vi "客户端侦听列表.vi"() -> ()   [LabVIEW 2016, in "wxpusher.lvlib"]
uses:
  wxpusher.lvlib
  <vilib>/Utility/miscctls.llb/LVPointTypeDef.ctl
  <vilib>/httpClient/LabVIEWHTTPClient.lvlib
panel:
  out "回调时间":timestamp
  out "有效主机列表":T1(array[cluster])
  out "长度":i32
  out "现场主机回调信息":string
  in  "开机启动":bool
  out "remote port":u16
  out "remote address":string
  out "服务器回调信息源码":string
  out "回调信息":T2
  out "新增主机列表":T1(array[cluster])
  in  "客户端列表":i32(listbox)
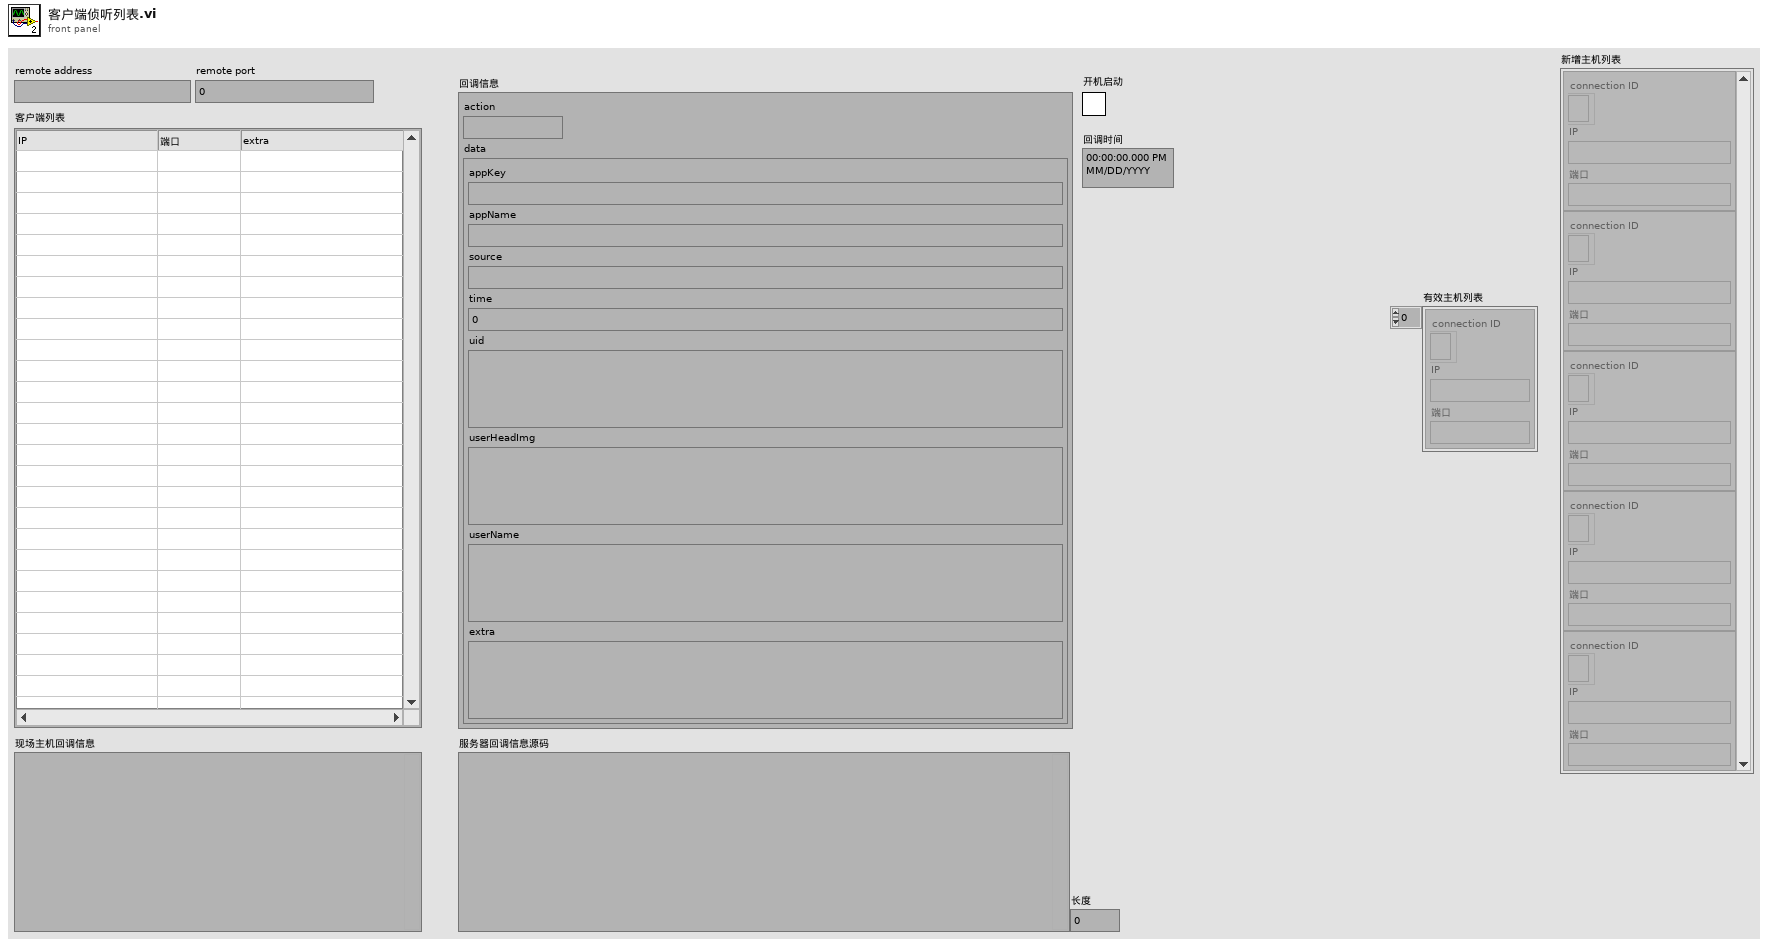
[diagram p1: front panel]
types:
  T1 = cluster{"connection ID":refnum<k5>, "IP":string, "端口":string}[]
  T2 = cluster{"action":string, "data":cluster{"appKey":string, "appName":string, "source":string, "time":u64, "uid":string, "userHeadImg":string, "userName":string, "extra":string}}
  T3 = typedef "LVPointTypeDef.ctl" = cluster{"Horizontal":i16, "Vertical":i16}
  T4 = cluster{"数据输出":string, "data":cluster{"action":string, "data":cluster{"appKey":string, "appName":string, "source":string, "time":u64, "uid":string, "userHeadImg":string, "userName":string, "extra":string}}}
  T5 = cluster{"connection ID":refnum<k5>, "IP":string, "端口":string}
  T6 = enum16{"Standard", "Buffered", "CRLF", "Immediate"}
  T7 = cluster{"cmd":string, "data":cluster{"png":u8[]}}
  T8 = typedef "LabVIEWHTTPClient.lvlib/ClientHandle.ctl" = refnum<k1>
  T9 = cluster{"data out":string, "类型和默认值":cluster{"action":string, "data":cluster{"appKey":string, "appName":string, "source":string, "time":u64, "uid":string, "userHeadImg":string, "userName":string, "extra":string}}}
  T10 = cluster{"cmd":string, "data":cluster{"action":string, "data":cluster{"appKey":string, "appName":string, "source":string, "time":u64, "uid":string, "userHeadImg":string, "userName":string, "extra":string}}}
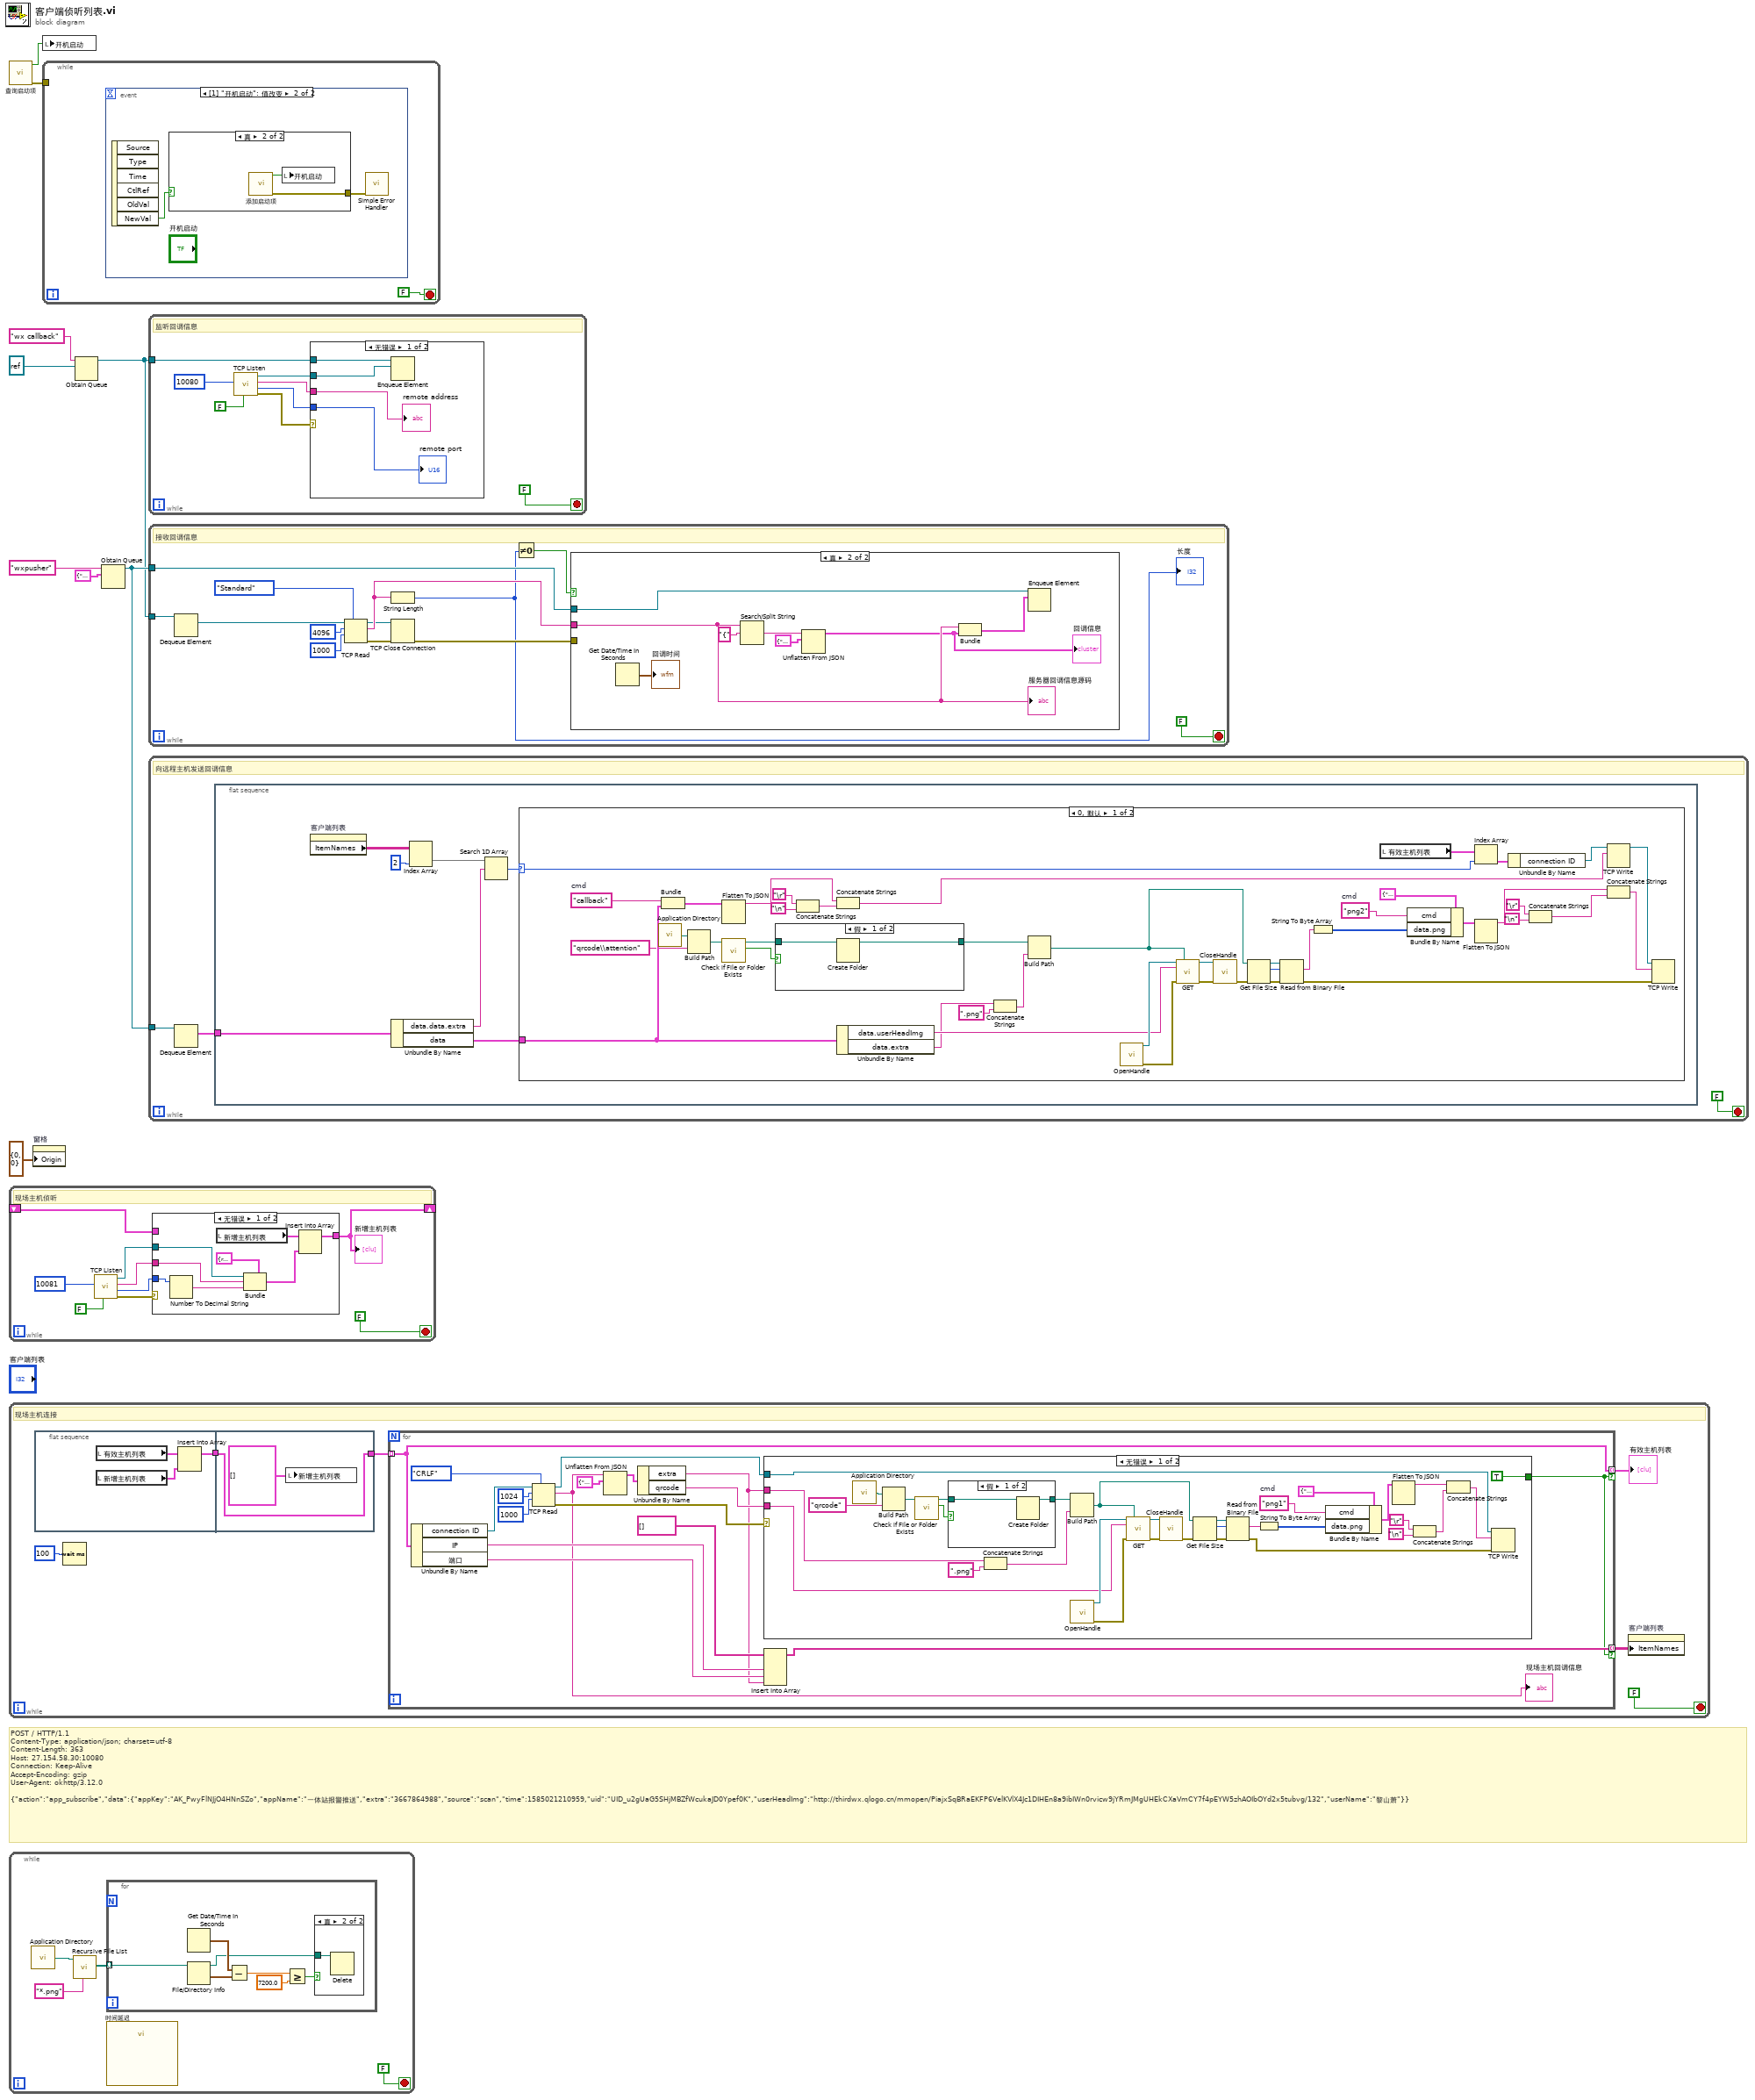
[diagram p0: block diagram]
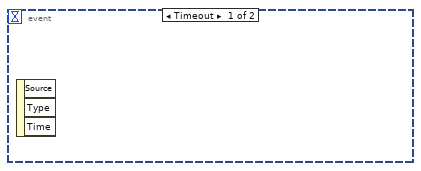
[diagram p3: hidden frame]
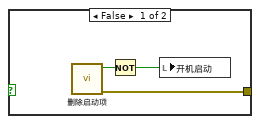
[diagram p4: hidden frame]
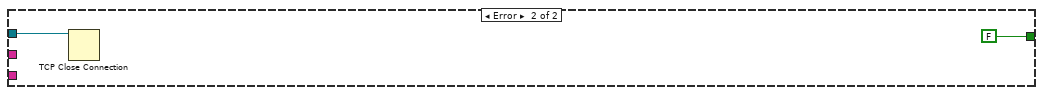
[diagram p10: hidden frame]
diagram:
  # "POST / HTTP/1.1\nContent-Type: application/json; charset=utf-8\nContent-Length: 363\nHost: 27.154.58.30:10080\nConnection: Keep-Alive\nAccept-Encoding: gzip\nUser-Agent: okhttp/3.12.0\n\n{\"action\":\"app_subscribe\",\"data\":{\"appKey\":\"AK_PwyFlNJjO4HNnSZo\",\"appName\":\"一体站报警推送\",\"extra\":\"3667864988\",\"source\":\"scan\",\"time\":1585021210959,\"uid\":\"UID_u2gUaG5SHjMBZfWcukaJD0Ypef0K\",\"userHeadImg\":\"http://thirdwx.qlogo.cn/mmopen/PiajxSqBRaEKFP6VelKVlX4Jc1DIHEn8a9ibIWn0rvicw9jYRmJMgUHEkCXaVmCY7f4pEYW5zhAOIbOYd2x5tubvg/132\",\"userName\":\"黎山萧\"}}"
  n1 = call "查询启动项.vi"() -> ("error out"=w6:errorcluster, "包含启动项"=w5:bool)  [unwired: 10 in]
  n2 = while {
    shift-right: [w12] -> _
    shift-left: _ -> [w11]
    stop <- FALSE stop-if-true
    # "现场主机侦听"
    n3 = call <vilib>:"TCP Listen.vi"("resolve remote address (T)"=FALSE, "port"=u16 10081) -> ("error out"=w16:errorcluster, "remote port"=w13:u16, "remote address"=w14:string, "connection ID"=w15:refnum<k5>)  [unwired: 5 in, 1 out]
    n4 = case shown="无错误" w16 {
      tunnel: w15 -> [w26 _]
      tunnel: w14 -> [w20 _]
      tunnel: w13 -> [w21 _]
      tunnel: [w24 w27] -> w12
      tunnel: w11 -> [_ w27]
      frame No Error {
        n5 = Number To Decimal String(number=w21) -> (decimal integer string=w23:string)  [unwired: 1 in]
        n6 = local read "新增主机列表"() -> (w19:T1)
        n7 = Bundle(cluster=T5 {"connection ID"=refnum, "IP"="", "端口"=""} ("簇"), "connection ID"=w26, "IP"=w20, "端口"=w23) -> (w25:T5)
        n8 = Insert Into Array(array=w19, new element=w25) -> (w24:T1)  [unwired: 1 in]
      }
      frame Error {
      }
    }
    "新增主机列表" <- w12
  }
  n9 = while {
    stop <- FALSE stop-if-true
    # "现场主机连接"
    n10 = flat-sequence {
      tunnel: [w34] -> w28
      tunnel: [w38] -> w30
      tunnel: w28 -> [w38]
      frame #0 {
        n11 = local read "有效主机列表"() -> (w35:T1)
        n12 = local read "新增主机列表"() -> (w36:T1)
        n13 = Insert Into Array(array=w35, new element=w36) -> (w34:T1)  [unwired: 1 in]
      }
      frame #1 {
        n14 = local write "新增主机列表"(T1 [] ("新增主机列表")) -> ()
      }
    }
    n15 = Wait (ms)(milliseconds to wait=u32 100 ("等待时间（毫秒）")) -> ()  [unwired: 1 out]
    n16 = for {
      tunnel: w30 -> [w44] mode=indexing
      tunnel: [w49] -> w31 mode=indexing if=w43
      tunnel: [w44] -> w29 mode=indexing if=w43
      n17 = Unbundle By Name(w44) -> ("connection ID"=w55:refnum<k5>, "IP"=w52:string, "端口"=w51:string)
      n18 = TCP Read(connection ID=w55, bytes to read=1024 ("读取的字节"), 7:T6."CRLF" ("模式（标准）"), 9:1000 ("超时毫秒(25000)")) -> (connection ID out=w42:refnum<k5>, data out=w47:string, error out=w48:errorcluster)  [unwired: 1 in]
      "现场主机回调信息" <- w47
      n19 = Unflatten From JSON(JSON string=w47, type and defaults=cluster{"extra":string, "qrcode":string} {"extra"="", "qrcode"=""}) -> (value=w45:cluster{"extra":string, "qrcode":string})  [unwired: 5 in, 1 out]
      n20 = Unbundle By Name(w45) -> ("extra"=w40:string, "qrcode"=w41:string)
      n21 = case shown="无错误" w48 {
        tunnel: [TRUE FALSE] -> w43
        tunnel: w42 -> [w58 w91]
        tunnel: w41 -> [w57 _]
        tunnel: w40 -> [w56 _]
        frame No Error {
          w84 = "png1"  # cmd
          n22 = call <vilib>:"Application Directory.vi"() -> ("Application Directory"=w76:path)
          n23 = Build Path(base path=w76, name or relative path="qrcode" ("名称或相对路径")) -> (appended path=w64:path)
          n24 = call <vilib>:"Check if File or Folder Exists.vi"("path"=w64) -> ("file or folder exists?"=w66:bool, "dup path"=w65:path)  [unwired: 8 in, 1 out]
          n25 = case shown="假" w66 {
            tunnel: [w89 w90] -> w63
            tunnel: w65 -> [w88 w90]
            frame False {
              n26 = Create Folder(path (use dialog)=w88) -> (created path=w89:path)  [unwired: 2 in, 2 out]
            }
            frame True {
            }
          }
          n27 = Concatenate Strings(w56, ".png" ("字符串")) -> (w69:string)
          n28 = Build Path(base path=w63, name or relative path=w69) -> (appended path=w70:path)
          n29 = call <vilib>:"OpenHandle.vi"() -> ("client handle out"=w59:T8, "error out"=w60:errorcluster)  [unwired: 14 in]
          n30 = call <vilib>:"GET.vi"("client handle"=w59, "output file"=w70, "url"=w57, "error in (no error)"=w60) -> ("client handle out"=w61:T8, "error out"=w62:errorcluster)  [unwired: 8 in, 2 out]
          n31 = call <vilib>:"CloseHandle.vi"("client handle"=w61, "error in (no error)"=w62) -> ("error out"=w72:errorcluster)  [unwired: 13 in]
          n32 = Get File Size(file=w70, error in=w72) -> (refnum out=w71:refnum<file>, size (in bytes)=w74:i64, 0:w73:errorcluster)
          n33 = Read from Binary File(8:w73, 10:w74, 11:w71) -> (0:w75:errorcluster, 2:w85:string)  [unwired: 3 in, 2 out]
          n34 = String To Byte Array(string=w85) -> (unsigned byte array=w86:u8[])
          n35 = Bundle By Name(cluster=T7 {"cmd"="", "data"={"png"=[]}}, "cmd"=w84, "data.png"=w86) -> (w78:T7)
          n36 = Flatten To JSON(anything=w78) -> (JSON string=w79:string)  [unwired: 2 in, 1 out]
          n37 = Concatenate Strings("\r", "\n") -> (w83:string)
          n38 = Concatenate Strings(w79, w83) -> (w80:string)
          n39 = TCP Write(connection ID=w58, data in=w80, error in (no error)=w75) -> ()  [unwired: 1 in, 3 out]
        }
        frame Error {
          n40 = TCP Close Connection(connection ID=w91) -> ()  [unwired: 2 in, 2 out]
        }
      }
      n41 = Insert Into Array(array=string[] [] ("数组"), new element #1=w52, new element #2=w51, new element #3=w40) -> (w49:string[])  [unwired: 1 in]
    }
    "有效主机列表" <- w29
    n42 = property on="客户端列表" class="MCListbox (严格)"("ItemNames"=w31) -> ()  [unwired: 2 in, 2 out]
  }
  n43 = while {
    stop <- FALSE stop-if-true
    n44 = call <vilib>:"Application Directory.vi"() -> ("Application Directory"=w95:path)
    n45 = call <vilib>:"Recursive File List.vi"("pattern"="*.png", "Folder Path"=w95) -> ("All Files in Dir"=w93:path[])  [unwired: 5 in, 4 out]
    n46 = for {
      tunnel: w93 -> [w103] mode=indexing
      n47 = Get Date/Time In Seconds() -> (seconds since 1Jan1904=w101:timestamp)
      n48 = File/Directory Info(path=w103) -> (path out=w97:path, last mod=w102:timestamp)  [unwired: 1 in, 5 out]
      n49 = Subtract(x=w101, y=w102) -> (x-y=w100:dbl)
      n50 = Greater Or Equal?(x=w100, y=7200.0) -> (x >= y?=w98:bool)
      n51 = case shown="真" w98 {
        tunnel: w97 -> [_ w104]
        frame False {
        }
        frame True {
          n52 = Delete(path (use dialog)=w104) -> ()  [unwired: 4 in, 3 out]
        }
      }
    }
    n53 = call "时间延迟"() -> ()  [unwired: 11 in, 1 out]
  }
  n54 = property on="窗格" class="Pane"("Origin"=T3 {"Horizontal"=0, "Vertical"=0} ("原点")) -> ()  [unwired: 2 in, 2 out]
  n55 = local write "开机启动"(w5) -> ()
  n56 = while {
    tunnel: w6 -> [_]
    stop <- FALSE stop-if-true
    n57 = event shown="[1] \"开机启动\": 值改变" {
      selector: _ -> [_ _]
      dyn-events: _ -> [_ _]
      timeout: _ -> [_ _]
      event Timeout {
        n58 = event-data() -> ()  [unwired: 1 in, 3 out]
      }
      event "开机启动": Value Change {
        n59 = event-data() -> ("NewVal"=w107:bool)  [unwired: 1 in, 5 out]
        n60 = case shown="真" w107 {
          tunnel: [w108 w111] -> w106
          frame False {
            n61 = call "删除启动项.vi"() -> ("error out"=w108:errorcluster, "删除标记"=w110:bool)  [unwired: 10 in]
            n62 = Not(x=w110) -> (.not. x?=w109:bool)
            n63 = local write "开机启动"(w109) -> ()
          }
          frame True {
            n64 = call "添加启动项.vi"() -> ("error out"=w111:errorcluster, "添加成功标记"=w112:bool)  [unwired: 10 in]
            n65 = local write "开机启动"(w112) -> ()
          }
        }
        n66 = call <vilib>:"Simple Error Handler.vi"("error in (no error)"=w106) -> ()  [unwired: 4 in, 5 out]
      }
    }
  }
  n67 = Obtain Queue(name (unnamed)="wx callback" ("名称（未命名）"), element data type=refnum<k5> refnum ("connection ID")) -> (queue out=w1:refnum<queue>)  [unwired: 3 in, 2 out]
  n68 = Obtain Queue(name (unnamed)="wxpusher" ("名称（未命名）"), element data type=T4 {"数据输出"="", "data"={"action"="", "data"={"appKey"="", "appName"="", "source"="", "time"=0, "uid"="", "userHeadImg"="", "userName"="", "extra"=""}}}) -> (queue out=w7:refnum<queue>)  [unwired: 3 in, 2 out]
  n69 = while {
    tunnel: w1 -> [w113]
    stop <- FALSE stop-if-true
    # "监听回调信息"
    n70 = call <vilib>:"TCP Listen.vi"("resolve remote address (T)"=FALSE, "port"=u16 10080) -> ("error out"=w118:errorcluster, "remote port"=w114:u16, "remote address"=w117:string, "connection ID"=w116:refnum<k5>)  [unwired: 5 in, 1 out]
    n71 = case shown="无错误" w118 {
      tunnel: w116 -> [w121 _]
      tunnel: w117 -> [w124 _]
      tunnel: w114 -> [w123 _]
      tunnel: w113 -> [w122 _]
      frame No Error {
        n72 = Enqueue Element(queue=w122, element=w121) -> ()  [unwired: 2 in, 3 out]
        "remote address" <- w124
        "remote port" <- w123
      }
      frame Error {
      }
    }
  }
  n73 = while "While循环" {
    tunnel: w7 -> [w136]
    tunnel: w1 -> [w131]
    stop <- FALSE stop-if-true
    # "接收回调信息"
    n74 = Dequeue Element(queue=w131) -> (element=w130:refnum<k5>)  [unwired: 2 in, 3 out]
    n75 = TCP Read(connection ID=w130, bytes to read=4096 ("读取的字节"), 7:T6."Standard" ("模式（标准）"), 9:1000 ("超时毫秒(25000)")) -> (connection ID out=w129:refnum<k5>, data out=w132:string, error out=w128:errorcluster)  [unwired: 1 in]
    n76 = String Length(string=w132) -> (length=w126:i32)
    "长度" <- w126
    n77 = TCP Close Connection(connection ID=w129, error in (no error)=w128) -> (error out=w127:errorcluster)  [unwired: 1 in, 1 out]
    n78 = Not Equal To 0?(x=w126) -> (x != 0?=w125:bool)
    n79 = case shown="真" w125 {
      tunnel: w136 -> [_ w145]
      tunnel: w132 -> [_ w144]
      tunnel: w127 -> [_ _]
      frame False {
      }
      frame True {
        n80 = Get Date/Time In Seconds() -> (seconds since 1Jan1904=→"回调时间":timestamp)
        n81 = Search/Split String(string=w144, search string/char (-)="{" ("搜索字符串/字符(-)")) -> (match + rest of string=w141:string)  [unwired: 1 in, 2 out]
        n82 = Unflatten From JSON(JSON string=w141, type and defaults=T2 {"action"="", "data"={"appKey"="", "appName"="", "source"="", "time"=0, "uid"="", "userHeadImg"="", "userName"="", "extra"=""}} ("类型和默认值")) -> (value=w140:T2)  [unwired: 5 in, 1 out]
        "回调信息" <- w140
        n83 = Bundle("data out"=w144, "类型和默认值"=w140) -> (w139:T9)  [unwired: 1 in]
        n84 = Enqueue Element(queue=w145, element=w139) -> ()  [unwired: 2 in, 3 out]
        "服务器回调信息源码" <- w144
      }
    }
  }
  n85 = while {
    tunnel: w7 -> [w148]
    stop <- FALSE stop-if-true
    # "向远程主机发送回调信息"
    n86 = Dequeue Element(queue=w148) -> (element=w146:T4)  [unwired: 2 in, 3 out]
    n87 = flat-sequence {
      tunnel: w146 -> [w155]
      frame #0 {
        n88 = property on="客户端列表" class="MCListbox (严格)"() -> ("ItemNames"=w154:string[][])  [unwired: 2 in, 2 out]
        n89 = Unbundle By Name(w155) -> ("data.data.extra"=w151:string, "data"=w149:T2)
        n90 = Index Array(array=w154, index (col)=2 ("禁用的索引 (列)")) -> (element=w152:string[])  [unwired: 1 in]
        n91 = Search 1D Array(1D array=w152, element=w151) -> (index of element=w150:i32)  [unwired: 1 in]
        n92 = case shown="0, 默认" w150 {
          selector: w150 -> [w197 _]
          tunnel: w149 -> [w189 _]
          frame 0, Default {
            w161 = "png2"  # cmd
            w188 = "callback"  # cmd
            n93 = call <vilib>:"Application Directory.vi"() -> ("Application Directory"=w169:path)
            n94 = Bundle("cmd"=w188, "data"=w189) -> (w187:T10)  [unwired: 1 in]
            n95 = Build Path(base path=w169, name or relative path="qrcode\\attention" ("名称或相对路径")) -> (appended path=w181:path)
            n96 = Flatten To JSON(anything=w187) -> (JSON string=w194:string)  [unwired: 2 in, 1 out]
            n97 = call <vilib>:"Check if File or Folder Exists.vi"("path"=w181) -> ("file or folder exists?"=w179:bool, "dup path"=w180:path)  [unwired: 8 in, 1 out]
            n98 = case shown="假" w179 {
              tunnel: [w200 w201] -> w182
              tunnel: w180 -> [w199 w201]
              frame False {
                n99 = Create Folder(path (use dialog)=w199) -> (created path=w200:path)  [unwired: 2 in, 2 out]
              }
              frame True {
              }
            }
            n100 = Concatenate Strings("\r", "\n") -> (w190:string)
            n101 = Concatenate Strings(w194, w190) -> (w193:string)
            n102 = Unbundle By Name(w189) -> ("data.userHeadImg"=w158:string, "data.extra"=w157:string)
            n103 = Concatenate Strings(w157, ".png" ("字符串")) -> (w176:string)
            n104 = Build Path(base path=w182, name or relative path=w176) -> (appended path=w175:path)
            n105 = call <vilib>:"OpenHandle.vi"() -> ("client handle out"=w186:T8, "error out"=w185:errorcluster)  [unwired: 14 in]
            n106 = call <vilib>:"GET.vi"("client handle"=w186, "output file"=w175, "url"=w158, "error in (no error)"=w185) -> ("client handle out"=w184:T8, "error out"=w183:errorcluster)  [unwired: 8 in, 2 out]
            n107 = call <vilib>:"CloseHandle.vi"("client handle"=w184, "error in (no error)"=w183) -> ("error out"=w173:errorcluster)  [unwired: 13 in]
            n108 = Get File Size(file=w175, error in=w173) -> (refnum out=w174:refnum<file>, size (in bytes)=w171:i64, 0:w172:errorcluster)
            n109 = Read from Binary File(8:w172, 10:w171, 11:w174) -> (0:w170:errorcluster, 2:w160:string)  [unwired: 3 in, 2 out]
            n110 = String To Byte Array(string=w160) -> (unsigned byte array=w159:u8[])
            n111 = local read "有效主机列表"() -> (w198:T1)
            n112 = Bundle By Name(cluster=T7 {"cmd"="", "data"={"png"=[]}}, "cmd"=w161, "data.png"=w159) -> (w167:T7)
            n113 = Index Array(array=w198, index=w197) -> (element=w196:T5)
            n114 = Flatten To JSON(anything=w167) -> (JSON string=w166:string)  [unwired: 2 in, 1 out]
            n115 = Unbundle By Name(w196) -> ("connection ID"=w195:refnum<k5>)
            n116 = Concatenate Strings("\r", "\n") -> (w162:string)
            n117 = TCP Write(connection ID=w195, data in=w193) -> (connection ID out=w156:refnum<k5>)  [unwired: 2 in, 2 out]
            n118 = Concatenate Strings(w166, w162) -> (w165:string)
            n119 = TCP Write(connection ID=w156, data in=w165, error in (no error)=w170) -> ()  [unwired: 1 in, 3 out]
          }
          frame -1 {
          }
        }
      }
    }
  }
